vi "section_ident.vi"(9 "theta_min":dbl, 10 "theta_max":dbl, 11 "theta":dbl) -> (3 "section":i16)   [LabVIEW 2013]
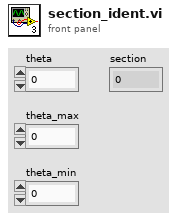
[diagram p1: front panel]
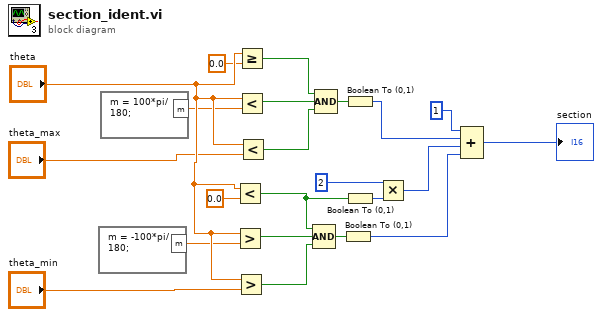
[diagram p0: block diagram]
diagram:
  n1 = formula code="m = -100*pi/180;"() -> ("m"=w12:dbl)
  n2 = formula code="m = 100*pi/180;"() -> ("m"=w2:dbl)
  n3 = Less?(x="theta", y=0.0) -> (x < y?=w15:bool)
  n4 = Greater?(x="theta", y=w12) -> (0:w10:bool)
  n5 = Greater?(x="theta", y="theta_min") -> (0:w9:bool)
  n6 = Greater Or Equal?(x="theta", y=0.0) -> (x >= y?=w4:bool)
  n7 = Less?(x="theta", y=w2) -> (x < y?=w5:bool)
  n8 = Less?(x="theta", y="theta_max") -> (x < y?=w6:bool)
  n9 = Compound Arithmetic op=AND(w15, w10, w9) -> (w8:bool)
  n10 = Compound Arithmetic op=AND(w4, w5, w6) -> (w7:bool)
  n11 = Boolean To (0,1)(Boolean=w8) -> (0, 1=w20:i16)
  n12 = Boolean To (0,1)(Boolean=w7) -> (0, 1=w18:i16)
  n13 = Boolean To (0,1)(Boolean=w15) -> (0, 1=w16:i16)
  n14 = Multiply(x=i16 2, y=w16) -> (x*y=w19:i16)
  n15 = Compound Arithmetic op=ADD(i16 1 ("value"), w18, w19, w20) -> (→"section":i16)
